vi "BP_hiddenLayer.vi"(4 "Weights_hX_IN":dbl[][](array[numeric]), 5 "Weights_outX(before being updated)":dbl[][](array[numeric]), 6 "Learning rate":dbl, 7 "Out_outX":dbl[](array[numeric]), 8 "Target_outX":dbl[](array[numeric]), 9 "Out_hx":dbl[](array[numeric]), 10 "Inputs":dbl[](array[numeric])) -> (2 "Weights_hX_OUT":dbl[][](array[numeric]))   [LabVIEW 2016]
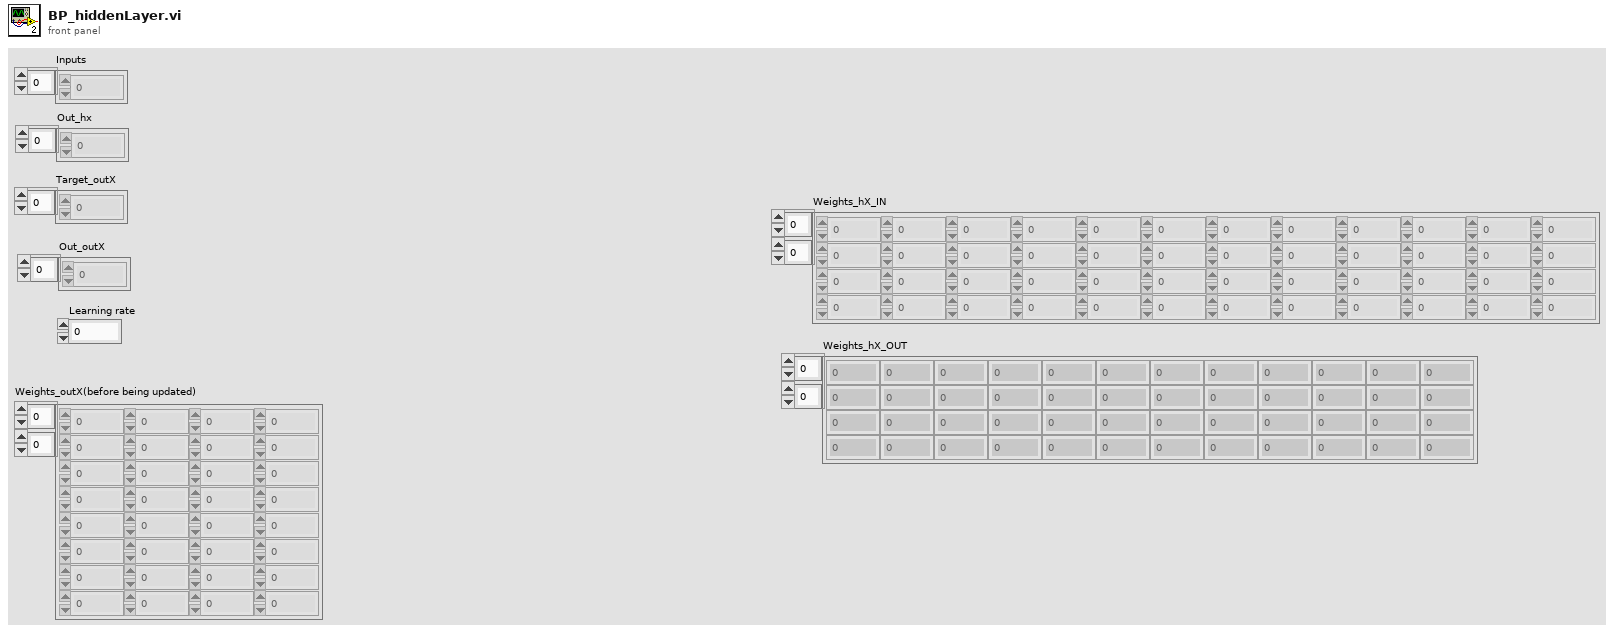
[diagram p1: front panel]
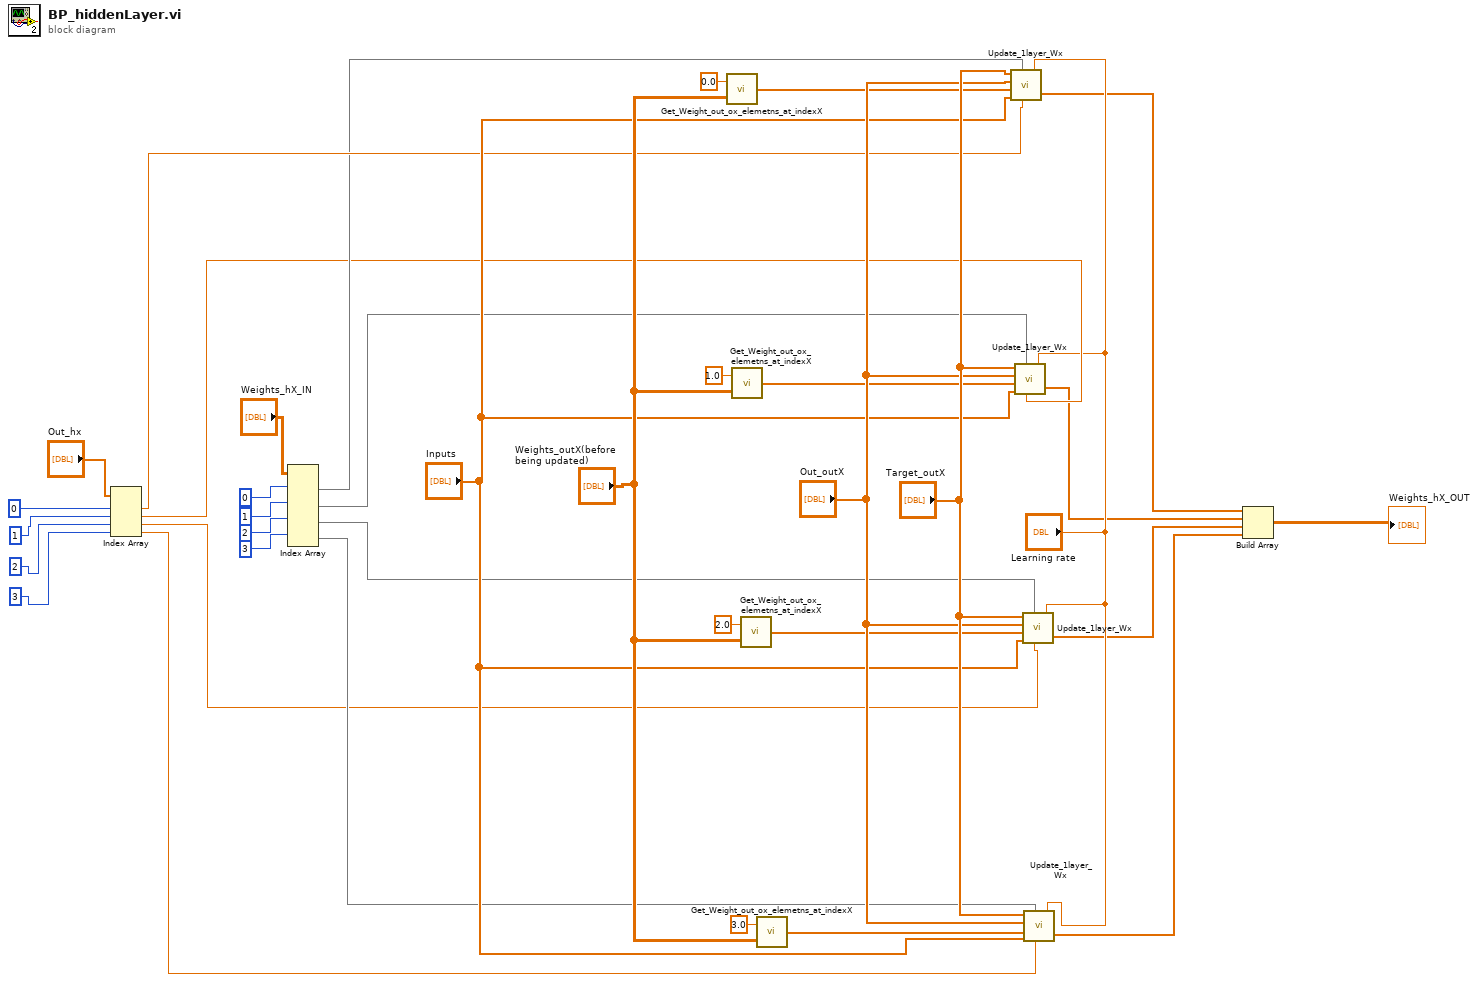
[diagram p0: block diagram]
diagram:
  n1 = Index Array(array="Out_hx", index #1=0 ("index"), index #2=1 ("index"), index #3=2 ("index"), index #4=3 ("index")) -> (element #1=w18:dbl, element #2=w13:dbl, element #3=w12:dbl, element #4=w11:dbl)
  n2 = Index Array(array="Weights_hX_IN", index (row) #1=0 ("index (row)"), index (row) #2=1 ("index (row)"), index (row) #3=2 ("index (row)"), index (row) #4=3 ("index (row)")) -> (element #1=w17:dbl[], element #2=w16:dbl[], element #3=w15:dbl[], element #4=w14:dbl[])  [unwired: 4 in]
  n3 = call "Get_Weight_out_ox_elemetns_at_indexX.vi"("Weights_outX(before being updated)"="Weights_outX(before being updated)", "Index"=0.0) -> ("Output_array"=w34:dbl[])
  n4 = call "Get_Weight_out_ox_elemetns_at_indexX.vi"("Weights_outX(before being updated)"="Weights_outX(before being updated)", "Index"=1.0) -> ("Output_array"=w33:dbl[])
  n5 = call "Get_Weight_out_ox_elemetns_at_indexX.vi"("Weights_outX(before being updated)"="Weights_outX(before being updated)", "Index"=2.0) -> ("Output_array"=w32:dbl[])
  n6 = call "Get_Weight_out_ox_elemetns_at_indexX.vi"("Weights_outX(before being updated)"="Weights_outX(before being updated)", "Index"=3.0) -> ("Output_array"=w31:dbl[])
  n7 = call "Update_1layer_Wx.vi"("Learning rate"="Learning rate", "1layer_Out_hx"=w18, "Array_Weights_hx"=w17, "Array_Inputs"="Inputs", "Array_2layer_Weights_at_Index_hx"=w34, "Array_Out_ox"="Out_outX", "Array_target_ox"="Target_outX") -> ("Array_Weights_hx_updated"=w8:dbl[])
  n8 = call "Update_1layer_Wx.vi"("Learning rate"="Learning rate", "1layer_Out_hx"=w13, "Array_Weights_hx"=w16, "Array_Inputs"="Inputs", "Array_2layer_Weights_at_Index_hx"=w33, "Array_Out_ox"="Out_outX", "Array_target_ox"="Target_outX") -> ("Array_Weights_hx_updated"=w7:dbl[])
  n9 = call "Update_1layer_Wx.vi"("Learning rate"="Learning rate", "1layer_Out_hx"=w12, "Array_Weights_hx"=w15, "Array_Inputs"="Inputs", "Array_2layer_Weights_at_Index_hx"=w32, "Array_Out_ox"="Out_outX", "Array_target_ox"="Target_outX") -> ("Array_Weights_hx_updated"=w6:dbl[])
  n10 = call "Update_1layer_Wx.vi"("Learning rate"="Learning rate", "1layer_Out_hx"=w11, "Array_Weights_hx"=w14, "Array_Inputs"="Inputs", "Array_2layer_Weights_at_Index_hx"=w31, "Array_Out_ox"="Out_outX", "Array_target_ox"="Target_outX") -> ("Array_Weights_hx_updated"=w5:dbl[])
  n11 = Build Array(w8, w7, w6, w5) -> (→"Weights_hX_OUT":dbl[][])
